vi "IDS_rt_ParametersHssl.vi"(8 "Error In":errorcluster, 9 "set?":bool, 10 "HsslParams Input":T1, 11 "deviceHandle":i32) -> (0 "Error Out":errorcluster, 2 "HsslParams Output":T1, 3 "deviceHandle out":i32)   [LabVIEW 2016]
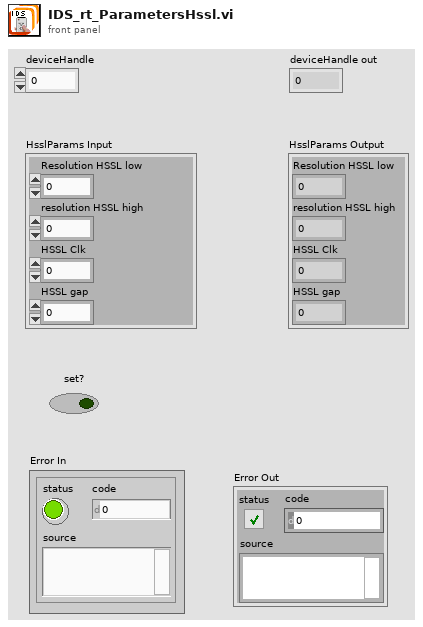
[diagram p1: front panel]
types:
  T1 = cluster{"Resolution HSSL low":i32, "resolution HSSL high":i32, "HSSL Clk ":i32, "HSSL gap":i32}
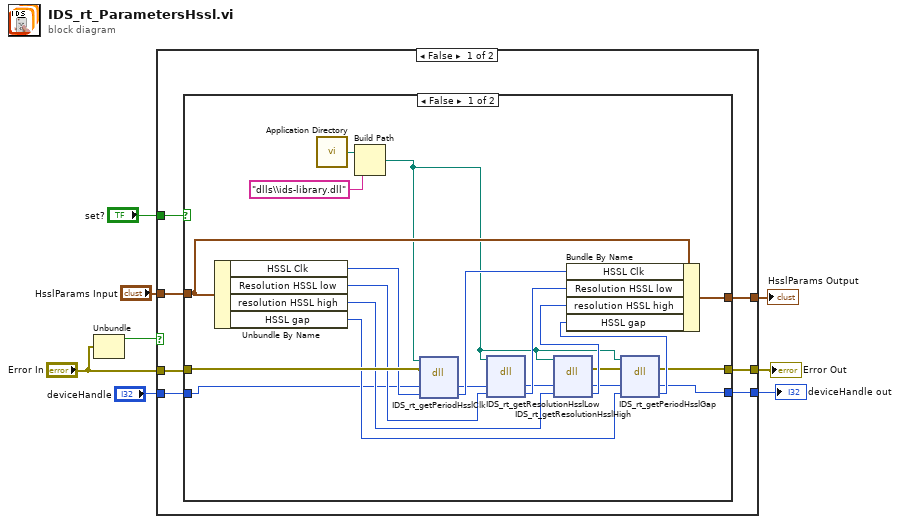
[diagram p0: block diagram]
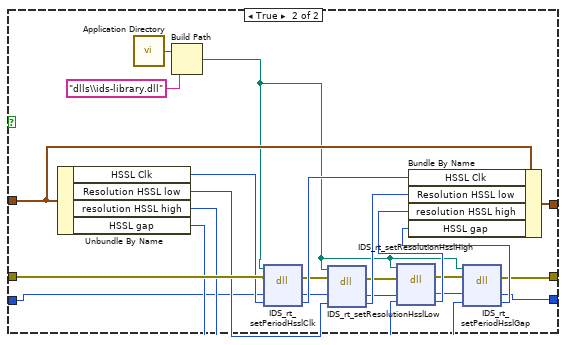
[diagram p2: hidden frame]
diagram:
  n1 = Unbundle("Error In") -> ("status"=w1:bool)  [unwired: 2 out]
  n2 = case shown="False" w1 {
    tunnel: "HsslParams Input" -> [w15 _]
    tunnel: [w13 w60] -> w7
    tunnel: "set?" -> [w14 _]
    tunnel: [w12 _] -> w3
    tunnel: [w11 w61] -> w5
    tunnel: "deviceHandle" -> [w10 w61]
    tunnel: "Error In" -> [w9 w60]
    frame False {
      n3 = case shown="False" w14 {
        tunnel: w15 -> [w36 w59]
        tunnel: w9 -> [w34 w57]
        tunnel: [w29 w52] -> w13
        tunnel: [w35 w58] -> w12
        tunnel: [w19 w40] -> w11
        tunnel: w10 -> [w23 w44]
        frame False {
          n4 = Unbundle By Name(w36) -> ("HSSL Clk"=w33:i32, "Resolution HSSL low"=w25:i32, "resolution HSSL high"=w28:i32, "HSSL gap"=w31:i32)
          n5 = call <vilib>:"Application Directory.vi"() -> ("Application Directory"=w18:path)
          n6 = Build Path(base path=w18, name or relative path="dlls\\ids-library.dll" ("ipAddress")) -> (appended path=w16:path)
          n7 = dll-call lib="C:/Users/matheus/Desktop/LabVIEW_Draft_V1.6.0/dlls/ids-library.*" fn="IDS_rt_getPeriodHsslClk"(path in=w16, error in=w34, "deviceHandle"=w23, "period"=w33) -> ("deviceHandle"=w22:i32, "period"=w32:i32)  [unwired: 2 in, 2 out]
          n8 = dll-call lib="C:/Users/matheus/Desktop/LabVIEW_Draft_V1.6.0/dlls/ids-library.*" fn="IDS_rt_getResolutionHsslLow"(path in=w16, "deviceHandle"=w22, "resolution"=w25) -> ("deviceHandle"=w21:i32, "resolution"=w24:i32)  [unwired: 3 in, 2 out]
          n9 = dll-call lib="C:/Users/matheus/Desktop/LabVIEW_Draft_V1.6.0/dlls/ids-library.*" fn="IDS_rt_getResolutionHsslHigh"(path in=w16, "deviceHandle"=w21, "resolution"=w28) -> (error out=w26:errorcluster, "deviceHandle"=w20:i32, "resolution"=w27:i32)  [unwired: 3 in, 1 out]
          n10 = dll-call lib="C:/Users/matheus/Desktop/LabVIEW_Draft_V1.6.0/dlls/ids-library.*" fn="IDS_rt_getPeriodHsslGap"(path in=w16, error in=w26, "deviceHandle"=w20, "gap"=w31) -> (error out=w29:errorcluster, "deviceHandle"=w19:i32, "gap"=w30:i32)  [unwired: 2 in, 1 out]
          n11 = Bundle By Name(cluster=w36, "HSSL Clk"=w32, "Resolution HSSL low"=w24, "resolution HSSL high"=w27, "HSSL gap"=w30) -> (w35:T1)
        }
        frame True {
          n12 = Unbundle By Name(w59) -> ("HSSL Clk"=w56:i32, "Resolution HSSL low"=w48:i32, "resolution HSSL high"=w51:i32, "HSSL gap"=w54:i32)
          n13 = call <vilib>:"Application Directory.vi"() -> ("Application Directory"=w39:path)
          n14 = Build Path(base path=w39, name or relative path="dlls\\ids-library.dll" ("ipAddress")) -> (appended path=w37:path)
          n15 = dll-call lib="C:/Users/matheus/Desktop/LabVIEW_Draft_V1.6.0/dlls/ids-library.*" fn="IDS_rt_setPeriodHsslClk"(path in=w37, error in=w57, "deviceHandle"=w44, "period"=w56) -> (error out=w46:errorcluster, "deviceHandle"=w43:i32, "period"=w55:i32)  [unwired: 2 in, 1 out]
          n16 = dll-call lib="C:/Users/matheus/Desktop/LabVIEW_Draft_V1.6.0/dlls/ids-library.*" fn="IDS_rt_setResolutionHsslLow"(path in=w37, error in=w46, "deviceHandle"=w43, "resolution"=w48) -> (error out=w45:errorcluster, "deviceHandle"=w42:i32, "resolution"=w47:i32)  [unwired: 2 in, 1 out]
          n17 = dll-call lib="C:/Users/matheus/Desktop/LabVIEW_Draft_V1.6.0/dlls/ids-library.*" fn="IDS_rt_setResolutionHsslHigh"(path in=w37, error in=w45, "deviceHandle"=w42, "resolution"=w51) -> (error out=w49:errorcluster, "deviceHandle"=w41:i32, "resolution"=w50:i32)  [unwired: 2 in, 1 out]
          n18 = dll-call lib="C:/Users/matheus/Desktop/LabVIEW_Draft_V1.6.0/dlls/ids-library.*" fn="IDS_rt_setPeriodHsslGap"(path in=w37, error in=w49, "deviceHandle"=w41, "gap"=w54) -> (error out=w52:errorcluster, "deviceHandle"=w40:i32, "gap"=w53:i32)  [unwired: 2 in, 1 out]
          n19 = Bundle By Name(cluster=w59, "HSSL Clk"=w55, "Resolution HSSL low"=w47, "resolution HSSL high"=w50, "HSSL gap"=w53) -> (w58:T1)
        }
      }
    }
    frame True {
    }
  }
  "Error Out" <- w7
  "deviceHandle out" <- w5
  "HsslParams Output" <- w3
